vi "pr_mod_v0.vi"() -> ()   [LabVIEW 2009]
panel:
  in  "stop":bool
  out "Viteza":dbl(knob)=50.97374767507157 scale=0.0..150.0
  in  "Viteza maxima":dbl(slide)=114.0 scale=0.0..150.0
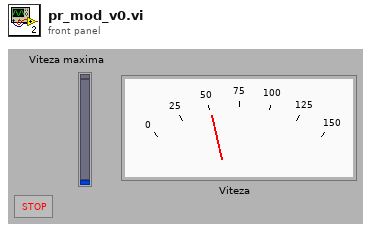
[diagram p1: front panel]
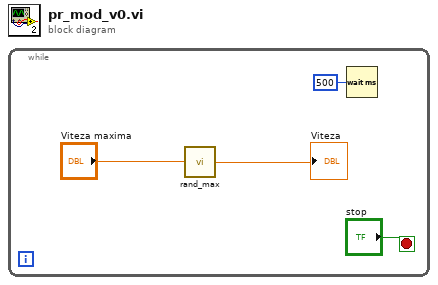
[diagram p0: block diagram]
diagram:
  n1 = while {
    stop <- "stop" stop-if-true
    n2 = call "rand_max.vi"("Val_max"="Viteza maxima") -> ("Val_out"=→"Viteza":dbl)
    n3 = Wait (ms)(milliseconds to wait=u32 500) -> ()  [unwired: 1 out]
  }
